vi "Connection.vi"(8 "error in":errorcluster) -> (0 "error out":errorcluster, 3 "Session Out":T1)   [LabVIEW 2015]
uses:
  <vilib>/userdefined/High Color/VBAIInterface.ctl
  <vilib>/vision/Vision Builder AI/API.llb/IVB Interface - VBAI Version.ctl
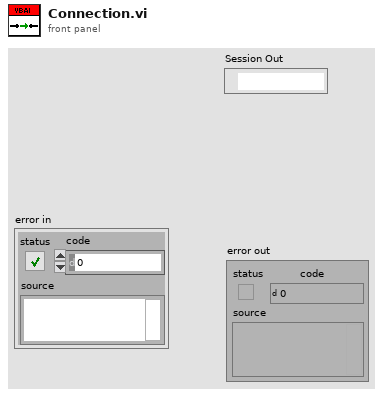
[diagram p1: front panel]
types:
  T1 = typedef "VBAIInterface.ctl" = refnum<k21>
  T2 = typedef "IVB Interface - VBAI Version.ctl" = u16
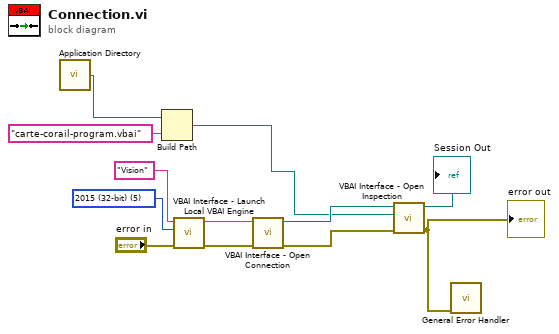
[diagram p0: block diagram]
diagram:
  w12 = T2 5 items=["2010 (32-bit)"=0, "2011 (32-bit)"=1, "2012 (32-bit)"=2, "2013 (32-bit)"=3, "2014 (32-bit)"=4, "2014 (64-bit)"=1004, "2015 (32-bit)"=5, "2015 (64-bit)"=1005] ("Engine Version")
  n1 = call <vilib>:"Application Directory.vi"() -> ("Application Directory"=w3:path)
  n2 = Build Path(base path=w3, name or relative path="carte-corail-program.vbai") -> (appended path=w1:path)
  n3 = call <vilib>:"VBAI Interface - Launch Local VBAI Engine.vi"("error in"="error in", "Engine Version"=w12, "Local VBAI Engine Name"="Vision") -> ("error out"=w9:errorcluster, "Session Name Out"=w10:string)  [unwired: 7 in]
  n4 = call <vilib>:"VBAI Interface - Open Connection.vi"("error in"=w9, "Session In"=w10) -> ("error out"=w7:errorcluster, "Session Out"=w8:T1)  [unwired: 8 in]
  n5 = call <vilib>:"VBAI Interface - Open Inspection.vi"("error in"=w7, "Path"=w1, "Session In"=w8) -> ("error out"=w5:errorcluster, "Session Out"=→"Session Out":T1)  [unwired: 7 in]
  "error out" <- w5
  n6 = call <vilib>:"General Error Handler.vi"("error in (no error)"=w5) -> ()  [unwired: 10 in, 5 out]
